vi "Populate Tree Ctl from Bucket.vi"(8 "error in (no error)":errorcluster, 9 "Tree Ctl Ref":refnum<vi>, 11 "Data.S3":refnum<class "Data.S3.lvclass">) -> (0 "error out":errorcluster, 1 "Tree Ctl Ref":refnum<vi>, 2 "Objects in bucket":T1[](array[typedef]), 3 "Data.S3 out":refnum<class "Data.S3.lvclass">, 4 "Common Prefixes":string[](array[string]))   [LabVIEW 2020, in "Data.S3.lvclass"]
uses:
  Data.S3.lvclass
  <vilib>/AWS Toolkit/S3/Object Content.ctl
  <vilib>/AWS Toolkit/S3/Storage Class.ctl
  <vilib>/AWS Toolkit/S3/Owner.ctl
  <vilib>/AWS Toolkit/S3/NI_AWS_S3.lvlib
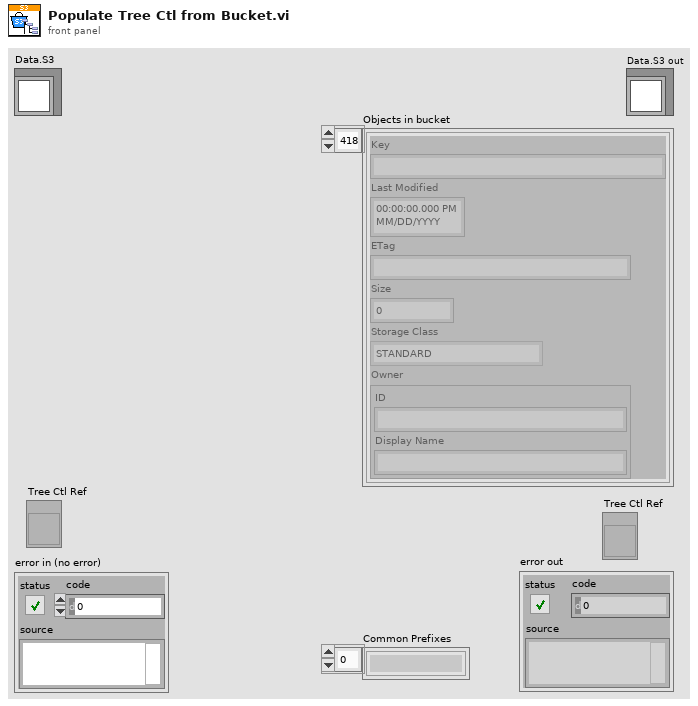
[diagram p1: front panel]
types:
  T1 = typedef "NI_AWS_S3.lvlib/Object Content.ctl" = cluster{"Key":string, "Last Modified":timestamp, "ETag":string, "Size":u64, "Storage Class":T2, "Owner":T3}
  T2 = typedef "NI_AWS_S3.lvlib/Storage Class.ctl" = enum16{"STANDARD", "REDUCED_REDUNDANCY"}
  T3 = typedef "NI_AWS_S3.lvlib/Owner.ctl" = cluster{"ID":string, "Display Name":string}
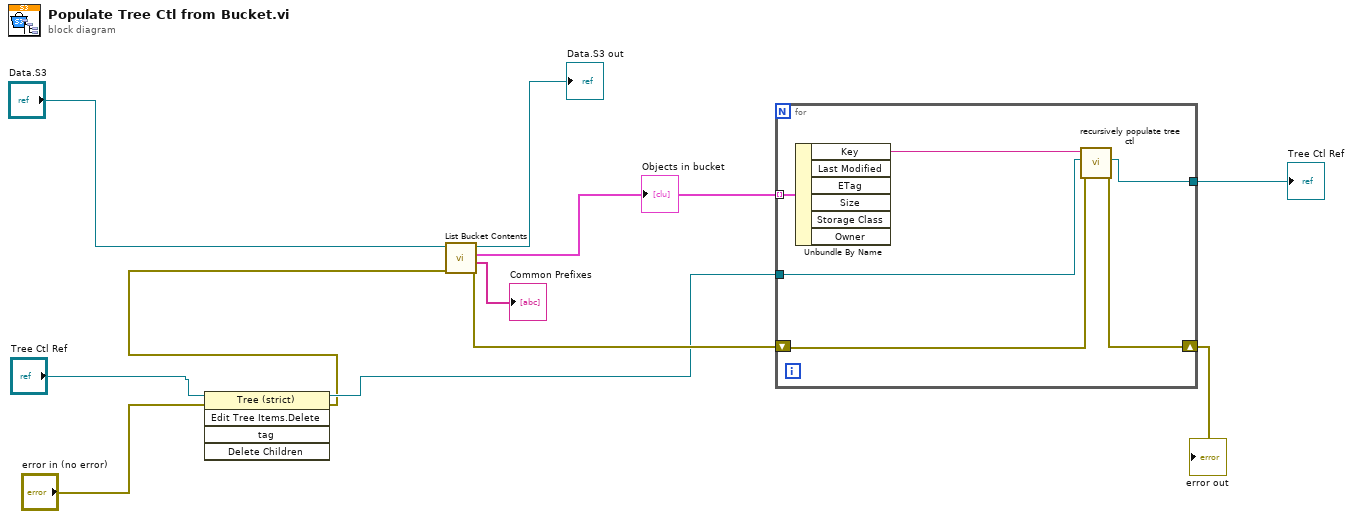
[diagram p0: block diagram]
diagram:
  n1 = invoke class="Tree (strict)" method="Edit Tree Items.Delete"(reference="Tree Ctl Ref", error in="error in (no error)") -> (reference out=w4:refnum<vi>, error out=w1:errorcluster)  [unwired: 3 in, 3 out]
  n2 = call "List Bucket Contents.vi"("error in (no error)"=w1, "Data.S3"="Data.S3") -> ("error out"=w8:errorcluster, "Common Prefixes"=→"Common Prefixes":string[], "Objects in bucket"=w10:T1[], "Data.S3 out"=→"Data.S3 out":refnum<class "Data.S3.lvclass">)  [unwired: 6 in]
  "Objects in bucket" <- w10
  n3 = for {
    tunnel: w10 -> [w17] mode=indexing
    tunnel: w4 -> [w15]
    shift-right: [w13] -> w7
    shift-left: w8 -> [w14]
    tunnel: [w12] -> w6
    n4 = Unbundle By Name(w17) -> ("Key"=w16:string)  [unwired: 5 out]
    n5 = call "recursively populate tree ctl.vi"("error in (no error)"=w14, "tree ctl ref"=w15, "Object path"=w16) -> ("error out"=w13:errorcluster, "reference out"=w12:refnum<vi>)  [unwired: 7 in]
  }
  "error out" <- w7
  "Tree Ctl Ref" <- w6
